vi "FileIO-Get Hierarchical Preset Parameter File.vi"(0 "Presets":refnum<vi>, 7 "folder":path) -> (4 "Name":string, 8 "selected":path)   [LabVIEW 2020]
uses:
  Controls/KMultilevel Ring/KMultilevel Ring.xctl
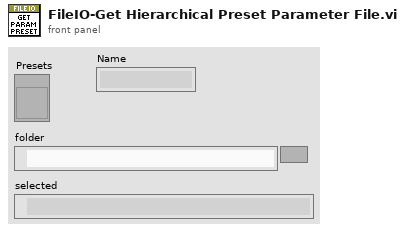
[diagram p1: front panel]
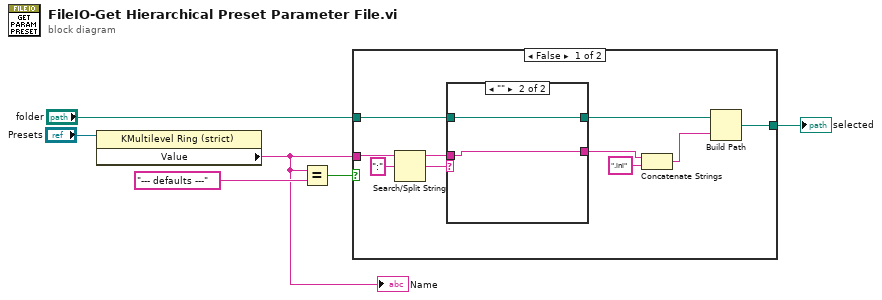
[diagram p0: block diagram]
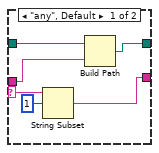
[diagram p2: hidden frame]
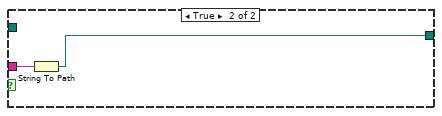
[diagram p3: hidden frame]
diagram:
  n1 = property on="Property Node" class="KMultilevel Ring (strict)"(reference="Presets") -> ("Value"=w4:string)  [unwired: 1 in, 2 out]
  "Name" <- w4
  n2 = Equal?(x=w4, y="--- defaults ---") -> (x = y?=w5:bool)
  n3 = case shown="False" w5 {
    tunnel: w4 -> [w13 w26]
    tunnel: [w15 w25] -> w2
    tunnel: "folder" -> [w9 _]
    frame False {
      n4 = Search/Split String(string=w13, search string/char (-)=":") -> (substring before match=w11:string, match + rest of string=w8:string)  [unwired: 1 in, 1 out]
      n5 = case shown="\"\"" w8 {
        selector: w8 -> [w19 _]
        tunnel: [w21 w24] -> w10
        tunnel: w9 -> [w22 w24]
        tunnel: [w17 w23] -> w7
        tunnel: w11 -> [w20 w23]
        frame "any", Default {
          n6 = String Subset(string=w19, offset (0)=1) -> (substring=w17:string)  [unwired: 1 in]
          n7 = Build Path(base path=w22, name or relative path=w20) -> (appended path=w21:path)
        }
        frame "" {
        }
      }
      n8 = Concatenate Strings(w7, ".ini" ("string")) -> (w14:string)
      n9 = Build Path(base path=w10, name or relative path=w14) -> (appended path=w15:path)
    }
    frame True {
      n10 = String To Path(string=w26) -> (path=w25:path)
    }
  }
  "selected" <- w2
